vi "constructCommand.vi"(6 "Time Stamp":timestamp, 8 "error in (no error)":errorcluster, 9 "svValue":variant, 10 "svArrayIndex":i32, 11 "DataListenerThisComponent in":refnum<class "DataListenerThisComponent.lvclass">) -> (0 "error out":errorcluster, 1 "validIsTrue":bool, 2 "command":refnum<class "Command.lvclass">, 3 "DataListenerThisComponent out":refnum<class "DataListenerThisComponent.lvclass">)   [LabVIEW 2012, in "DataListenerThisComponent.lvclass"]
doc: "Turns received shared variable information (from SubDataSVs) into commands (for the Command SV)."
uses:
  DataListenerThisComponent.lvclass
  C/Program Files (x86)/National Instruments/LabVIEW 2012/user.lib/Common/ComponentModel/ComponentModel/Command/Command.lvclass
  DataListenerThisComponent.lvclass/DataListenerThisComponent.ctl
  Typedefs/CommandValue.ctl
  ICommandFactory/ICommandFactory.lvclass
  C/Program Files (x86)/National Instruments/LabVIEW 2012/user.lib/Common/ComponentModel/ComponentModel/DataListener/DataListener.lvclass
  Typedefs/EXATypedefs.lvlib
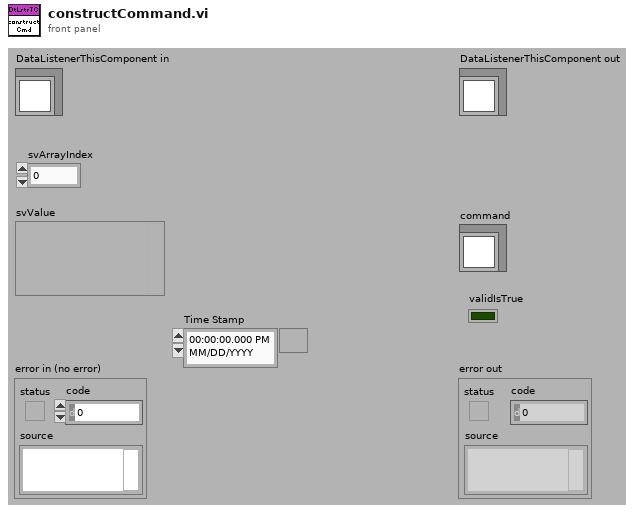
[diagram p1: front panel]
types:
  T1 = typedef "EXATypedefs.lvlib/SubDataSV.ctl" = enum16{"ClearError", "Disable", "Enable", "Exit", "GoToStandby", "HeartbeatIn", "Start"}
  T2 = typedef "EXATypedefs.lvlib/CommandValue.ctl" = enum16{"ClearError", "Disable", "Enable", "Exit", "GoToStandby", "OnHeartbeat", "OnIncomingMessagingError", "OnInterrupt", "Start"}
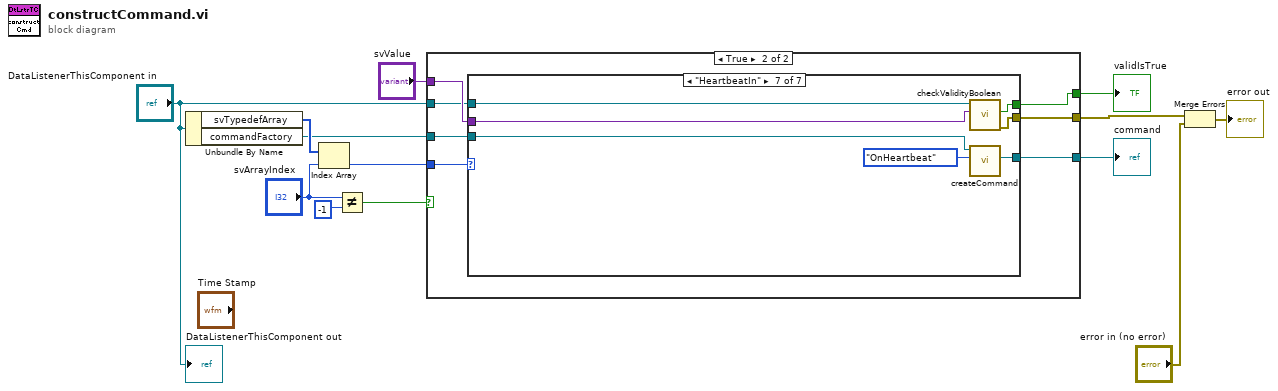
[diagram p0: block diagram]
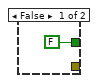
[diagram p2: hidden frame]
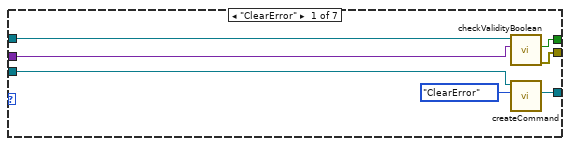
[diagram p3: hidden frame]
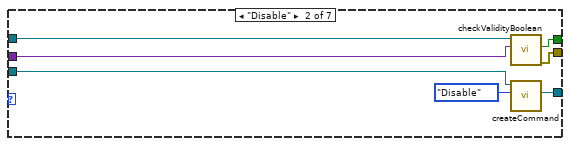
[diagram p4: hidden frame]
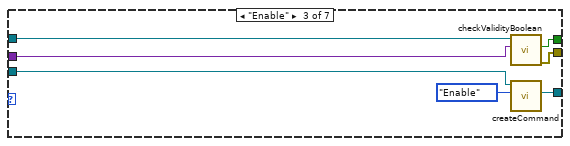
[diagram p5: hidden frame]
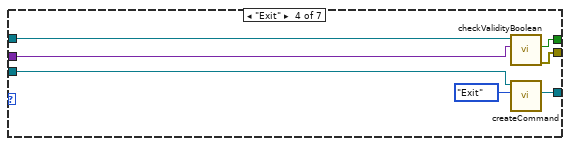
[diagram p6: hidden frame]
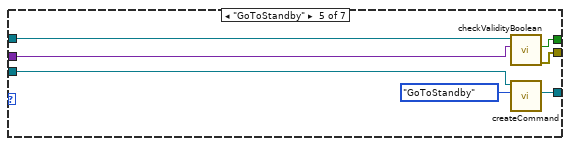
[diagram p7: hidden frame]
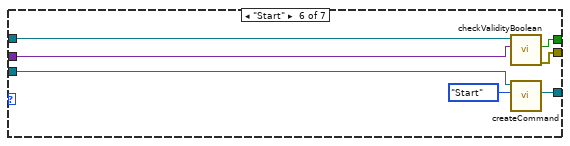
[diagram p8: hidden frame]
diagram:
  n1 = Unbundle By Name("DataListenerThisComponent in") -> ("svTypedefArray"=w7:T1[], "commandFactory"=w1:refnum<class "ICommandFactory.lvclass">)
  n2 = Index Array(array=w7, index="svArrayIndex") -> (element=w5:T1)
  n3 = Not Equal?(x="svArrayIndex", y=-1) -> (x != y?=w3:bool)
  n4 = case shown="True" w3 {
    tunnel: [_ w21] -> w8
    tunnel: "svValue" -> [_ w20]
    tunnel: [_ w19] -> w6
    tunnel: w5 -> [_ w18]
    tunnel: [FALSE w17] -> w2
    tunnel: "DataListenerThisComponent in" -> [_ w16]
    tunnel: w1 -> [_ w15]
    frame False {
    }
    frame True {
      n5 = case shown="\"HeartbeatIn\"" w18 {
        tunnel: [w22 w29 w36 w43 w50 w57 w64] -> w21
        tunnel: w20 -> [w27 w34 w41 w48 w55 w62 w69]
        tunnel: [w25 w32 w39 w46 w53 w60 w67] -> w19
        tunnel: [w26 w33 w40 w47 w54 w61 w68] -> w17
        tunnel: w16 -> [w28 w35 w42 w49 w56 w63 w70]
        tunnel: w15 -> [w23 w30 w37 w44 w51 w58 w65]
        frame "ClearError" {
          n6 = call "checkValidityBoolean.vi"("svValue"=w27, "DataListener in"=w28) -> ("error out"=w25:errorcluster, "validIsTrue"=w26:bool)  [unwired: 7 in, 1 out]
          n7 = call-dynamic "createCommand.vi"("commandValue"=CommandValue."ClearError", "ICommandFactory in"=w23) -> ("command"=w22:refnum<class "Command.lvclass">)  [unwired: 7 in, 2 out]
        }
        frame "Disable" {
          n8 = call "checkValidityBoolean.vi"("svValue"=w34, "DataListener in"=w35) -> ("error out"=w32:errorcluster, "validIsTrue"=w33:bool)  [unwired: 7 in, 1 out]
          n9 = call-dynamic "createCommand.vi"("commandValue"=CommandValue."Disable", "ICommandFactory in"=w30) -> ("command"=w29:refnum<class "Command.lvclass">)  [unwired: 7 in, 2 out]
        }
        frame "Enable" {
          n10 = call "checkValidityBoolean.vi"("svValue"=w41, "DataListener in"=w42) -> ("error out"=w39:errorcluster, "validIsTrue"=w40:bool)  [unwired: 7 in, 1 out]
          n11 = call-dynamic "createCommand.vi"("commandValue"=CommandValue."Enable", "ICommandFactory in"=w37) -> ("command"=w36:refnum<class "Command.lvclass">)  [unwired: 7 in, 2 out]
        }
        frame "Exit" {
          n12 = call "checkValidityBoolean.vi"("svValue"=w48, "DataListener in"=w49) -> ("error out"=w46:errorcluster, "validIsTrue"=w47:bool)  [unwired: 7 in, 1 out]
          n13 = call-dynamic "createCommand.vi"("commandValue"=CommandValue."Exit", "ICommandFactory in"=w44) -> ("command"=w43:refnum<class "Command.lvclass">)  [unwired: 7 in, 2 out]
        }
        frame "GoToStandby" {
          n14 = call "checkValidityBoolean.vi"("svValue"=w55, "DataListener in"=w56) -> ("error out"=w53:errorcluster, "validIsTrue"=w54:bool)  [unwired: 7 in, 1 out]
          n15 = call-dynamic "createCommand.vi"("commandValue"=CommandValue."GoToStandby", "ICommandFactory in"=w51) -> ("command"=w50:refnum<class "Command.lvclass">)  [unwired: 7 in, 2 out]
        }
        frame "Start" {
          n16 = call "checkValidityBoolean.vi"("svValue"=w62, "DataListener in"=w63) -> ("error out"=w60:errorcluster, "validIsTrue"=w61:bool)  [unwired: 7 in, 1 out]
          n17 = call-dynamic "createCommand.vi"("commandValue"=CommandValue."Start", "ICommandFactory in"=w58) -> ("command"=w57:refnum<class "Command.lvclass">)  [unwired: 7 in, 2 out]
        }
        frame "HeartbeatIn" {
          n18 = call "checkValidityBoolean.vi"("svValue"=w69, "DataListener in"=w70) -> ("error out"=w67:errorcluster, "validIsTrue"=w68:bool)  [unwired: 7 in, 1 out]
          n19 = call-dynamic "createCommand.vi"("commandValue"=CommandValue."OnHeartbeat", "ICommandFactory in"=w65) -> ("command"=w64:refnum<class "Command.lvclass">)  [unwired: 7 in, 2 out]
        }
      }
    }
  }
  "command" <- w8
  "validIsTrue" <- w2
  n20 = Merge Errors(w6, "error in (no error)") -> (→"error out":errorcluster)
  "DataListenerThisComponent out" <- "DataListenerThisComponent in"
